vi "Pre Launch Init.vi"(11 "Interlock in":refnum<class "Interlock.lvclass">) -> (0 "error out":errorcluster, 3 "Interlock out":refnum<class "Interlock.lvclass">)   [LabVIEW 2015, in "Interlocks.lvlib" / "Interlock.lvclass"]
doc: "(<B>Filename</B>: Actor Framework.lvlib:Actor.lvclass:Pre Launch Init.vi)\n\nDefines behavior that occurs after the Launch Nested Actor method is invoked but before the actor's Actor Core method begins running.\n\nBy default, this method does nothing. A descendant class may override it to define behavior."
uses:
  Interlock.lvclass
  <vilib>/ActorFramework/Actor/Actor.lvclass/Actor.ctl
  <vilib>/ActorFramework/Message Enqueuer/Message Enqueuer.lvclass/Message Enqueuer.ctl
  Interlock.lvclass/Interlock.ctl
  <vilib>/ActorFramework/Message Enqueuer/Init from Existing Queue.vi
  <vilib>/ActorFramework/Actor/Actor.lvclass
  <vilib>/ActorFramework/Message Enqueuer/Message Enqueuer.lvclass
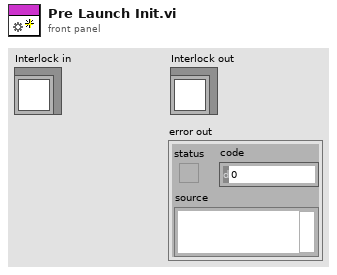
[diagram p1: front panel]
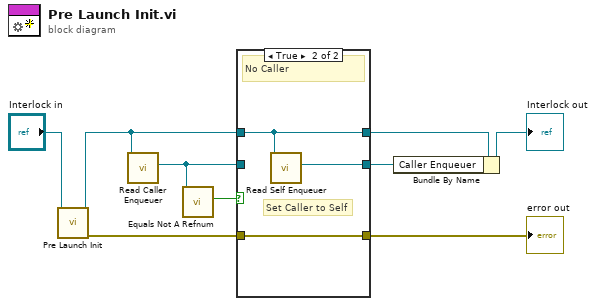
[diagram p0: block diagram]
diagram:
  n1 = call-parent "Pre Launch Init.vi"("Actor in"="Interlock in") -> ("error out"=w8:errorcluster, "Actor out"=w7:refnum<class "Interlock.lvclass">)  [unwired: 9 in]
  n2 = call <vilib>:"Read Caller Enqueuer.vi"("Actor"=w7) -> ("Caller Enqueuer"=w2:refnum<class "Message Enqueuer.lvclass">)  [unwired: 10 in]
  n3 = call <vilib>:"Equals Not A Refnum.vi"("Message Enqueuer"=w2) -> ("Not a refnum?"=w1:bool)  [unwired: 10 in]
  n4 = case shown="True" w1 {
    tunnel: w8 -> [w11 w15]
    tunnel: w7 -> [w12 w14]
    tunnel: [w11 w15] -> w6
    tunnel: [w12 w14] -> w5
    tunnel: [w10 w13] -> w3
    tunnel: w2 -> [w10 _]
    frame False {
    }
    frame True {
      # "Set Caller to Self"
      # "No Caller"
      n5 = call <vilib>:"Read Self Enqueuer.vi"("Actor"=w14) -> ("Self Enqueuer"=w13:refnum<class "Message Enqueuer.lvclass">)  [unwired: 10 in]
    }
  }
  "error out" <- w6
  n6 = Bundle By Name(cluster=w5, "Caller Enqueuer"=w3) -> (→"Interlock out":refnum<class "Interlock.lvclass">)
